vi "io_bin_data_instrument_to_PCfile.vi"(7 "Target PC file":path, 8 "error in":errorcluster, 10 "Query (none)":string, 11 "VISA resource name":refnum<visa-resource-name>) -> (0 "error out":errorcluster, 1 "Data Size":i64, 3 "VISA resource name out":refnum<visa-resource-name>)   [LabVIEW 2014, in "rszvl_rsidr_core.lvlib"]
uses:
  rszvl_rsidr_core.lvlib
  type_Error_Codes.ctl
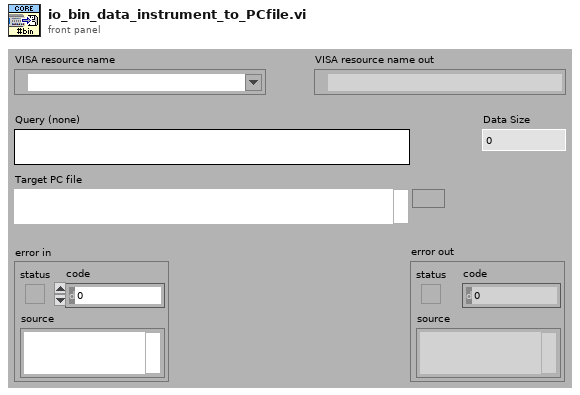
[diagram p1: front panel]
types:
  T1 = typedef "rszvl_rsidr_core.lvlib/type_Error_Codes.ctl" = enum16{"No_error", "VISA_err_ResourceNotFound", "VISA_err_Timeout", "VISA_warn_MoreDataAvailable", "RS_err_MissingCallback", "RS_err_InvalidAttribute", "RS_err_InvalidValue", "RS_err_UnknownResource", "RS_err_AlreadyInitialized", "RS_err_InstrumentStatus", "RS_err_BadRepCapName", "RS_err_TypesMismatch", "RS_err_ValueNotSupported", "RS_err_InvalidRngTable", "RS_err_IDqueryFail", "RS_err_UnexpResponse", "VISA_warn_ConfigNotLoaded", "RS_err_AttributeNotReadable", "RS_err_AttributeNotWritable", "RS_err_InstrumentType", "RS_err_InstrumentOption", "VISA_err_InvalidSize", "RS_err_ReliabilityIndicator", "VISA_warn_UnknownStatus", "VISA_warn_TermCharRead", "VISA_err_IO_error"}
  T2 = enum16{"open", "replace", "create", "open or create", "replace or create", "replace or create with confirmation"}
  T3 = typedef "rszvl_rsidr_core.lvlib/type_Session_Data.ctl" = cluster{"Instr type":string, "Instr type for err. msg.":string, "Installed Options":string[], "OPC Timeout":i32, "Query Instrument Status":bool, "Check Range":bool, "Check Options":bool, "Add LF to Write":bool, "Simulate":bool, "Logging":bool, "Logging params":variant, "Interface Type":enum16{"Unknown", "GPIB", "VXI", "GPIB_VXI", "ASRL", "PXI", "TCPIP", "USB", "SOCKET"}, "Fast Sweep":i32, "AdditionalFlags":i32, "WaitBeforeWrite":i32, "WaitBeforeRead":i32, "BinDataChunkSize":i64}
  T4 = enum16{"Unknown", "GPIB", "VXI", "GPIB_VXI", "ASRL", "PXI", "TCPIP", "USB", "SOCKET"}
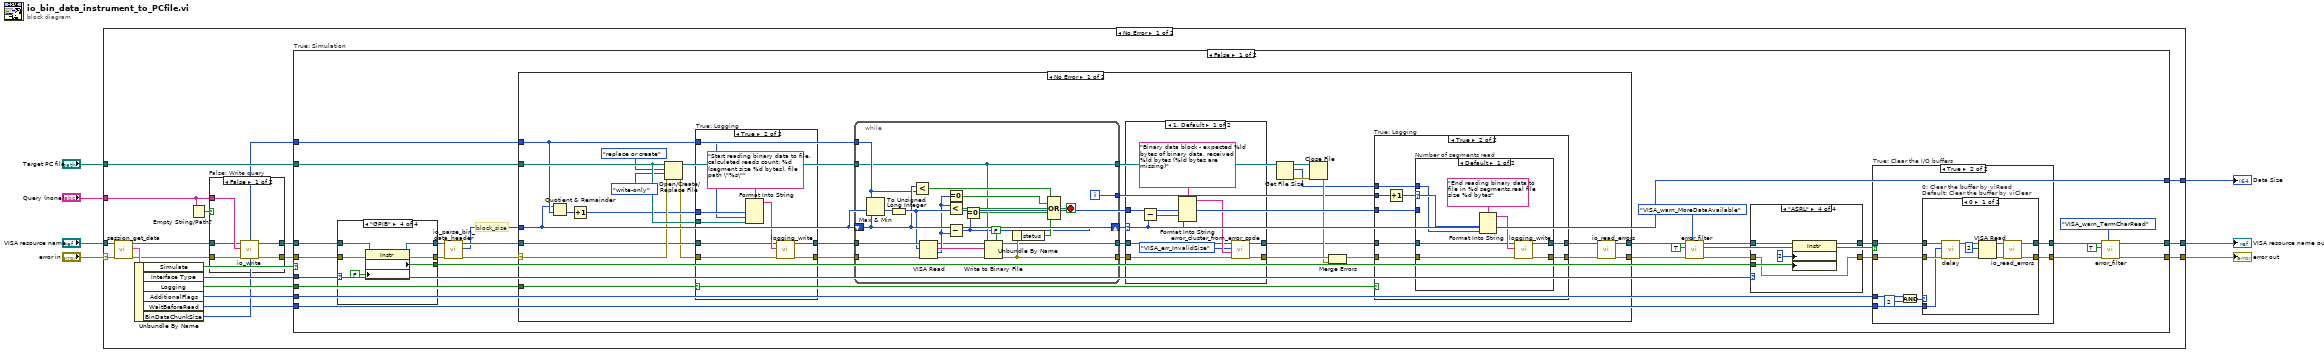
[diagram p0: block diagram]
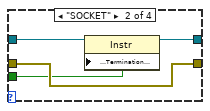
[diagram p4: hidden frame]
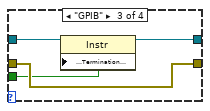
[diagram p5: hidden frame]
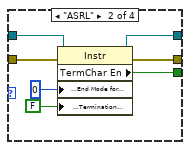
[diagram p7: hidden frame]
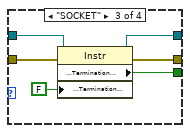
[diagram p8: hidden frame]
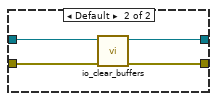
[diagram p10: hidden frame]
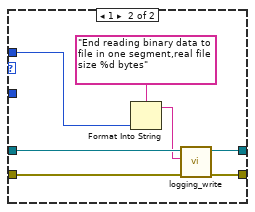
[diagram p12: hidden frame]
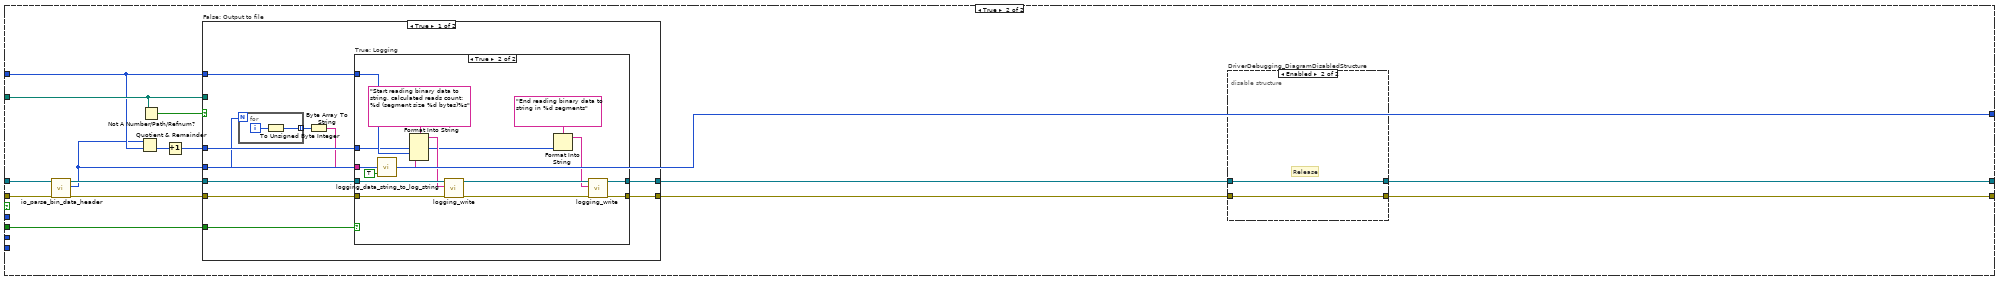
[diagram p16: hidden frame]
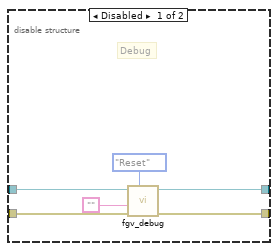
[diagram p17: hidden frame]
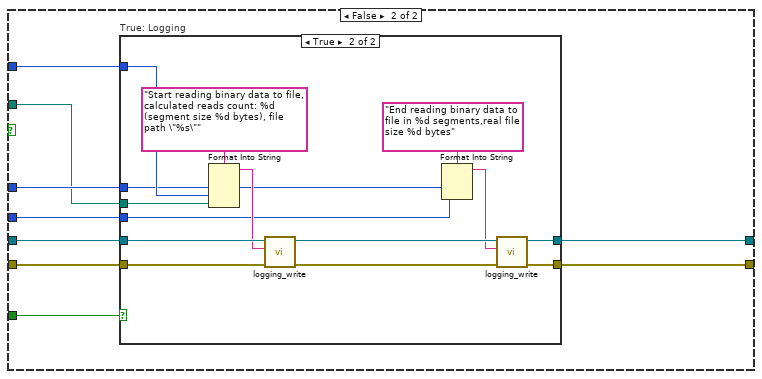
[diagram p19: hidden frame]
diagram:
  n1 = case shown="No Error" "error in" {
    selector: "error in" -> [w23 w302]
    tunnel: "Target PC file" -> [w26 _]
    tunnel: [w25 w301] -> w6
    tunnel: [w24 w302] -> w5
    tunnel: "VISA resource name" -> [w22 w301]
    tunnel: "Query (none)" -> [w12 _]
    tunnel: [w8 _] -> w1
    frame No Error {
      n2 = call "session_get_data.vi"("error in"=w23, "VISA resource name"=w22) -> ("error out"=w16:errorcluster, "Session User Data out"=w20:T3, "VISA resource name out"=w15:refnum<visa-resource-name>)  [unwired: 7 in]
      n3 = Unbundle By Name(w20) -> ("Simulate"=w21:bool, "Interface Type"=w19:T4, "Logging"=w18:bool, "AdditionalFlags"=w11:i32, "WaitBeforeRead"=w9:i32, "BinDataChunkSize"=w10:i64)
      n4 = Empty String/Path?(string/path=w12) -> (empty?=w17:bool)
      n5 = case "False: Write query" shown="False" w17 {
        tunnel: w16 -> [w30 w32]
        tunnel: [w28 w32] -> w14
        tunnel: [w27 w33] -> w13
        tunnel: w12 -> [w31 _]
        tunnel: w15 -> [w29 w33]
        frame False {
          n6 = call "io_write.vi"("error in"=w30, "write buffer"=w31, "VISA resource name"=w29) -> ("error out"=w28:errorcluster, "VISA resource name out"=w27:refnum<visa-resource-name>)  [unwired: 7 in]
        }
        frame True {
        }
      }
      n7 = case "True: Simulation" shown="False" w21 {
        tunnel: w14 -> [w50 w234]
        tunnel: w13 -> [w51 w235]
        tunnel: w26 -> [w62 w236]
        tunnel: [w40 w225] -> w25
        tunnel: [w39 w226] -> w24
        tunnel: w19 -> [w54 _]
        tunnel: w18 -> [w53 w238]
        tunnel: w10 -> [w52 w231]
        tunnel: w11 -> [w49 _]
        tunnel: w9 -> [w35 _]
        tunnel: [w34 w224] -> w8
        frame False {
          # "block_size"
          n8 = case "4: ASRL" shown="\"GPIB\"" w54 {
            tunnel: w50 -> [w78 w85 w92 w98]
            tunnel: w51 -> [w79 w84 w91 w97]
            tunnel: [w79 w83 w90 w96] -> w57
            tunnel: [w78 w82 w89 w95] -> w58
            tunnel: [_ w80 w87 w93] -> w38
            frame Default {
            }
            frame "ASRL" {
              n9 = property on="Property Node" class="Instr"(reference=w84, error in=w85, "Serial Settings:End Mode for Reads"=u16 0 ("ASRL End In"), "Message Based Settings:Termination Character Enable"=FALSE ("TermChar En")) -> (reference out=w83:refnum<visa-resource-name>, error out=w82:errorcluster, "TermChar En"=w80:bool)
            }
            frame "SOCKET" {
              n10 = property on="Property Node" class="Instr"(reference=w91, error in=w92, "Message Based Settings:Termination Character Enable"=FALSE ("TermChar En")) -> (reference out=w90:refnum<visa-resource-name>, error out=w89:errorcluster, "Message Based Settings:Termination Character Enable"=w87:bool)
            }
            frame "GPIB" {
              n11 = property on="Property Node" class="Instr"(reference=w97, error in=w98, "Message Based Settings:Termination Character Enable"=FALSE ("TermChar En")) -> (reference out=w96:refnum<visa-resource-name>, error out=w95:errorcluster, "Message Based Settings:Termination Character Enable"=w93:bool)
            }
          }
          n12 = call "io_parse_bin_data_header.vi"("error in"=w58, "VISA resource name"=w57) -> ("error out"=w56:errorcluster, "Size of the bin data"=w34:i64, "VISA resource name out"=w55:refnum<visa-resource-name>)  [unwired: 6 in, 1 out]
          n13 = case shown="No Error" w56 {
            selector: w56 -> [w151 w223]
            tunnel: [w146 w223] -> w37
            tunnel: w55 -> [w150 w222]
            tunnel: w34 -> [w141 _]
            tunnel: w52 -> [w144 _]
            tunnel: w62 -> [w152 _]
            tunnel: [w145 w222] -> w36
            tunnel: w53 -> [w149 _]
            frame No Error {
              n14 = Quotient & Remainder(x=w141, y=w144) -> (floor(x/y)=w148:i64)  [unwired: 1 out]
              n15 = Increment(x=w148) -> (x+1=w147:i64)
              n16 = Open/Create/Replace File(file path (use dialog)=w152, error in=w151, operation (0:open)=T2."replace or create", access (0:read/write)=enum16{"read/write", "read-only", "write-only"}."write-only") -> (refnum out=w130:refnum<file>, error out=w138:errorcluster)  [unwired: 2 in, 1 out]
              n17 = case "True: Logging" shown="True" w149 {
                tunnel: w138 -> [w212 w221]
                tunnel: [w212 w220] -> w133
                tunnel: w150 -> [w211 w218]
                tunnel: [w211 w217] -> w134
                tunnel: w152 -> [_ w213]
                tunnel: w144 -> [_ w214]
                tunnel: w147 -> [_ w215]
                frame False {
                }
                frame True {
                  n18 = Format Into String(format string="Start reading binary data to file, calculated reads count: %d (segment size %d bytes), file path \"%s\"", w215, w214, w213) -> (resulting string=w219:string)  [unwired: 2 in, 1 out]
                  n19 = call "logging_write.vi"("error in"=w221, "String to write"=w219, "VISA resource name"=w218) -> ("error out"=w220:errorcluster, "VISA resource name out"=w217:refnum<visa-resource-name>)  [unwired: 7 in]
                }
              }
              n20 = while {
                tunnel: w133 -> [w196]
                tunnel: w134 -> [w198]
                tunnel: w144 -> [w186]
                shift-right: [w178] -> w135
                shift-left: w141 -> [w187]
                tunnel: [w192] -> w136
                tunnel: w130 -> [w184]
                tunnel: [w184] -> w124
                tunnel: [w183] -> w126
                tunnel: [w182] -> w137
                i -> [w183]
                stop <- w189 stop-if-true
                n21 = Max & Min(x=w186, y=w187) -> (min(x,y)=w197:i64)  [unwired: 1 out]
                n22 = To Unsigned Long Integer(number=w197) -> (unsigned 32bit integer=w193:u32)
                n23 = Less?(x=w187, y=w186) -> (x < y?=w185:bool)
                n24 = VISA Read(VISA resource name=w198, byte count=w193, error in (no error)=w196) -> (VISA resource name out=w182:refnum<visa-resource-name>, read buffer=w195:string, return count=w191:u32, error out=w194:errorcluster)
                n25 = Equal To 0?(x=w191) -> (x = 0?=w188:bool)
                n26 = Less?(x=w191, y=w193) -> (x < y?=w190:bool)
                n27 = Subtract(x=w187, y=w191) -> (x-y=w178:i64)
                n28 = Equal To 0?(x=w178) -> (x = 0?=w179:bool)
                n29 = Write to Binary File(file (use dialog)=w184, data=w195, error in=w194, 5:FALSE ("prepend array or string size? (T)")) -> (error out=w192:errorcluster)  [unwired: 2 in, 2 out]
                n30 = Unbundle By Name(w192) -> ("status"=w180:bool)
                n31 = Compound Arithmetic op=OR(w185, w188, w190, w179, w180) -> (w189:bool)
              }
              n32 = case shown="1, Default" w135 {
                selector: w135 -> [w203 _]
                tunnel: w136 -> [w206 w210]
                tunnel: [w207 w210] -> w129
                tunnel: w141 -> [w205 _]
                tunnel: w137 -> [w200 w209]
                tunnel: [w199 w209] -> w125
                frame 1, Default {
                  n33 = Subtract(x=w205, y=w203) -> (x-y=w204:i64)
                  n34 = Format Into String(format string="Binary data block - expected %ld bytes of binary data, received %ld bytes (%ld bytes are missing)" ("error message (\"\")"), w205, w204, w203) -> (resulting string=w202:string)  [unwired: 2 in, 1 out]
                  n35 = call "error_cluster_from_error_code.vi"("error in"=w206, "error message (\"\")"=w202, "Error Enum in"=type_Error_Codes."VISA_err_InvalidSize", "VISA resource name"=w200) -> ("error out"=w207:errorcluster, "VISA resource name out"=w199:refnum<visa-resource-name>)  [unwired: 6 in]
                }
                frame 0 {
                }
              }
              n36 = Get File Size(file=w124) -> (refnum out=w131:refnum<file>, size (in bytes)=w123:i64, 0:w132:errorcluster)  [unwired: 1 in]
              n37 = Close File(refnum=w131, error in=w132) -> (error out=w128:errorcluster)  [unwired: 1 out]
              n38 = Merge Errors(w129, w128) -> (w127:errorcluster)
              n39 = case "True: Logging" shown="True" w149 {
                tunnel: w125 -> [w153 w159]
                tunnel: w127 -> [w154 w160]
                tunnel: [w154 w158] -> w142
                tunnel: [w153 w157] -> w143
                tunnel: w126 -> [_ w162]
                tunnel: w141 -> [_ w156]
                tunnel: w123 -> [_ w155]
                frame False {
                }
                frame True {
                  n40 = Increment(x=w162) -> (x+1=w161:i32)
                  n41 = case "Number of segments read" shown="Default" w161 {
                    selector: w161 -> [w165 _]
                    tunnel: w160 -> [w169 w177]
                    tunnel: w159 -> [w168 w176]
                    tunnel: [w167 w175] -> w158
                    tunnel: [w166 w174] -> w157
                    tunnel: w156 -> [_ _]
                    tunnel: w155 -> [w164 w171]
                    frame Default {
                      n42 = Format Into String(format string="End reading binary data to file in %d segments,real file size %d bytes", w165, w164) -> (resulting string=w170:string)  [unwired: 2 in, 1 out]
                      n43 = call "logging_write.vi"("error in"=w169, "String to write"=w170, "VISA resource name"=w168) -> ("error out"=w167:errorcluster, "VISA resource name out"=w166:refnum<visa-resource-name>)  [unwired: 7 in]
                    }
                    frame 1 {
                      n44 = Format Into String(format string="End reading binary data to file in one segment,real file size %d bytes", w171) -> (resulting string=w172:string)  [unwired: 2 in, 1 out]
                      n45 = call "logging_write.vi"("error in"=w177, "String to write"=w172, "VISA resource name"=w176) -> ("error out"=w175:errorcluster, "VISA resource name out"=w174:refnum<visa-resource-name>)  [unwired: 7 in]
                    }
                  }
                }
              }
              n46 = call "io_read_errors.vi"("error in"=w142, "VISA resource name"=w143) -> ("error out"=w146:errorcluster, "VISA resource name out"=w145:refnum<visa-resource-name>)  [unwired: 8 in]
            }
            frame Error {
            }
          }
          n47 = call "error_filter.vi"("Error Enum in"=type_Error_Codes."VISA_warn_MoreDataAvailable" ("Code to detect"), "error in"=w37, "Clear detected code (F)"=TRUE ("Clear detected error (F)"), "VISA resource name"=w36) -> ("error out"=w47:errorcluster, "Code Detected"=w61:bool, "VISA resource name out"=w48:refnum<visa-resource-name>)  [unwired: 5 in]
          n48 = case "4: ASRL" shown="\"ASRL\"" w54 {
            tunnel: w48 -> [w64 w68 w72 w75]
            tunnel: [w64 w67 w71 w76] -> w46
            tunnel: w47 -> [w63 w66 w70 w73]
            tunnel: [w63 w66 w70 w73] -> w45
            tunnel: w38 -> [_ w65 w69 w74]
            frame Default {
            }
            frame "SOCKET" {
              n49 = property on="Property Node" class="Instr"(reference=w68, "Message Based Settings:Termination Character Enable"=w65) -> (reference out=w67:refnum<visa-resource-name>)  [unwired: 1 in, 1 out]
            }
            frame "GPIB" {
              n50 = property on="Property Node" class="Instr"(reference=w72, "Message Based Settings:Termination Character Enable"=w69) -> (reference out=w71:refnum<visa-resource-name>)  [unwired: 1 in, 1 out]
            }
            frame "ASRL" {
              n51 = property on="Property Node" class="Instr"(reference=w75, "Serial Settings:End Mode for Reads"=u16 2 ("ASRL End In"), "Message Based Settings:Termination Character Enable"=w74) -> (reference out=w76:refnum<visa-resource-name>)  [unwired: 1 in, 1 out]
            }
          }
          n52 = case "True: Clear the I/O buffers" shown="True" w61 {
            tunnel: [w99 w106] -> w41
            tunnel: w46 -> [w100 w107]
            tunnel: w45 -> [w99 w108]
            tunnel: [w100 w105] -> w42
            tunnel: w49 -> [_ w104]
            tunnel: w35 -> [_ w101]
            frame False {
            }
            frame True {
              n53 = And(x=w104, y=2 ("x")) -> (x .and. y?=w103:i32)
              n54 = case "0: Clear the buffer by viRead\nDefault: Clear the buffer by viClear" shown="0" w103 {
                tunnel: w108 -> [w113 w122]
                tunnel: w107 -> [w112 w121]
                tunnel: [w115 w120] -> w106
                tunnel: [w114 w119] -> w105
                tunnel: w101 -> [w109 _]
                frame 0 {
                  n55 = call "delay.vi"("error in"=w113, "Milliseconds to wait"=w109, "VISA resource name"=w112) -> ("error out"=w111:errorcluster, "VISA resource name out"=w110:refnum<visa-resource-name>)  [unwired: 7 in]
                  n56 = VISA Read ("Read the junk")(VISA resource name=w110, byte count=u32 2, error in (no error)=w111) -> (VISA resource name out=w116:refnum<visa-resource-name>, error out=w117:errorcluster)  [unwired: 2 out]
                  n57 = call "io_read_errors.vi"("error in"=w117, "VISA resource name"=w116) -> ("error out"=w115:errorcluster, "VISA resource name out"=w114:refnum<visa-resource-name>)  [unwired: 8 in]
                }
                frame Default {
                  n58 = call "io_clear_buffers.vi"("error in"=w122, "VISA resource name"=w121) -> ("error out"=w120:errorcluster, "VISA resource name out"=w119:refnum<visa-resource-name>)  [unwired: 8 in]
                }
              }
            }
          }
          n59 = call "error_filter.vi"("Error Enum in"=type_Error_Codes."VISA_warn_TermCharRead", "error in"=w41, "Clear detected code (F)"=TRUE, "VISA resource name"=w42) -> ("error out"=w39:errorcluster, "VISA resource name out"=w40:refnum<visa-resource-name>)  [unwired: 5 in, 1 out]
        }
        frame True {
          n60 = call "io_parse_bin_data_header.vi"("error in"=w234, "VISA resource name"=w235) -> ("error out"=w232:errorcluster, "Size of the bin data"=w224:i64, "VISA resource name out"=w233:refnum<visa-resource-name>)  [unwired: 6 in, 1 out]
          n61 = Quotient & Remainder(x=w224, y=w231) -> (floor(x/y)=w230:i64)  [unwired: 1 out]
          n62 = Not A Number/Path/Refnum?(number/path/refnum=w236) -> (NaN/Path/Refnum?=w237:bool)
          n63 = Increment(x=w230) -> (x+1=w229:i64)
          n64 = case "False: Output to file" shown="True" w237 {
            tunnel: w233 -> [w256 w284]
            tunnel: w232 -> [w255 w283]
            tunnel: [w254 w282] -> w227
            tunnel: [w253 w281] -> w228
            tunnel: w238 -> [w252 w280]
            tunnel: w231 -> [w251 w279]
            tunnel: w236 -> [_ w277]
            tunnel: w229 -> [w250 w278]
            tunnel: w224 -> [w249 w276]
            frame True {
              n65 = for {
                N: w249 -> [_]
                tunnel: [w257] -> w248 mode=indexing
                i -> [w258]
                n66 = To Unsigned Byte Integer(number=w258) -> (unsigned 8bit integer=w257:u8)
              }
              n67 = Byte Array To String(unsigned byte array=w248) -> (string=w247:string)
              n68 = case "True: Logging" shown="True" w252 {
                tunnel: w255 -> [w260 w275]
                tunnel: [w260 w267] -> w254
                tunnel: w256 -> [w259 w274]
                tunnel: [w259 w268] -> w253
                tunnel: w251 -> [_ w271]
                tunnel: w250 -> [_ w265]
                tunnel: w247 -> [_ w262]
                frame False {
                }
                frame True {
                  n69 = call "logging_data_string_to_log_string.vi"("Force binary format (F)"=TRUE, "Raw string to log"=w262) -> ("Result log string"=w263:string)  [unwired: 3 in]
                  n70 = Format Into String(format string="Start reading binary data to string, calculated reads count: %d (segment size %d bytes)%s", w265, w271, w263) -> (resulting string=w272:string)  [unwired: 2 in, 1 out]
                  n71 = call "logging_write.vi"("error in"=w275, "String to write"=w272, "VISA resource name"=w274) -> ("error out"=w269:errorcluster, "VISA resource name out"=w270:refnum<visa-resource-name>)  [unwired: 7 in]
                  n72 = Format Into String(format string="End reading binary data to string in %d segments", w265) -> (resulting string=w264:string)  [unwired: 2 in, 1 out]
                  n73 = call "logging_write.vi"("error in"=w269, "String to write"=w264, "VISA resource name"=w270) -> ("error out"=w267:errorcluster, "VISA resource name out"=w268:refnum<visa-resource-name>)  [unwired: 7 in]
                }
              }
            }
            frame False {
              n74 = case "True: Logging" shown="True" w280 {
                tunnel: w283 -> [w286 w300]
                tunnel: [w286 w292] -> w282
                tunnel: w284 -> [w285 w299]
                tunnel: [w285 w293] -> w281
                tunnel: w279 -> [_ w296]
                tunnel: w278 -> [_ w291]
                tunnel: w277 -> [_ w289]
                tunnel: w276 -> [_ w287]
                frame False {
                }
                frame True {
                  n75 = Format Into String(format string="Start reading binary data to file, calculated reads count: %d (segment size %d bytes), file path \"%s\"", w291, w296, w289) -> (resulting string=w297:string)  [unwired: 2 in, 1 out]
                  n76 = call "logging_write.vi"("error in"=w300, "String to write"=w297, "VISA resource name"=w299) -> ("error out"=w294:errorcluster, "VISA resource name out"=w295:refnum<visa-resource-name>)  [unwired: 7 in]
                  n77 = Format Into String(format string="End reading binary data to file in %d segments,real file size %d bytes", w291, w287) -> (resulting string=w290:string)  [unwired: 2 in, 1 out]
                  n78 = call "logging_write.vi"("error in"=w294, "String to write"=w290, "VISA resource name"=w295) -> ("error out"=w292:errorcluster, "VISA resource name out"=w293:refnum<visa-resource-name>)  [unwired: 7 in]
                }
              }
            }
          }
          n79 = disable-structure "DriverDebugging_DiagramDisabledStructure" shown="Enabled" {
            disable-tunnel: w227 -> [w243 w245]
            disable-tunnel: [w241 w245] -> w226
            disable-tunnel: w228 -> [w242 w246]
            disable-tunnel: [w240 w246] -> w225
            frame Disabled {
              # "Debug"
              n80 = call "fgv_debug.vi"("Operation"=enum16{"Reset", "ReadCommand", "SetCommand"}."Reset", "error in"=w243, "Command in"="" ("Empty String Constant"), "VISA resource name"=w242) -> ("error out"=w241:errorcluster, "VISA resource name out"=w240:refnum<visa-resource-name>)  [unwired: 6 in]
            }
            frame Enabled {
              # "Release"
            }
          }
        }
      }
    }
    frame Error {
    }
  }
  "error out" <- w5
  "VISA resource name out" <- w6
  "Data Size" <- w1
